vi "Find Child UIDs.vi"(7 "Actor in":refnum<class "Actor.lvclass">) -> (2 "Child UIDs":T1)   [LabVIEW 2025, in "jettl.lvlib"]
uses:
  jettl.lvlib
  Child UIDs.ctl
  Actor/Actor.lvclass
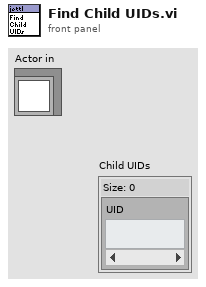
[diagram p1: front panel]
types:
  T1 = typedef "jettl.lvlib/Child UIDs.ctl" = set{string}
  T2 = typedef "jettl.lvlib/All Child Attributes.ctl" = map{string, refnum<class "Attributes.lvclass">}
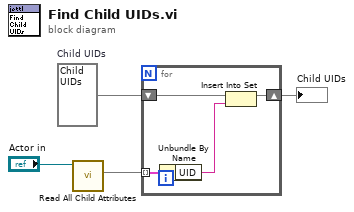
[diagram p0: block diagram]
diagram:
  w4 = T1 {}  # Child UIDs
  n1 = call-dynamic "Read All Child Attributes.vi"("Actor in"="Actor in") -> ("All Child Attributes"=w2:T2)  [unwired: 10 in]
  n2 = for {
    shift-right: [w7] -> w3
    shift-left: w4 -> [w8]
    tunnel: w2 -> [w5] mode=indexing
    n3 = Unbundle By Name(w5) -> ("UID"=w6:string)
    n4 = Insert Into Set(10:w6, 11:w8) -> (3:w7:T1)  [unwired: 1 out]
  }
  "Child UIDs" <- w3
